vi "enqueue.vi"(6 "priority (f)":bool, 8 "error in (no error)":errorcluster, 9 "data":variant, 10 "cmd":T1, 11 "ComicVine_manager in":refnum<class "ComicVine_manager.lvclass">) -> (0 "error out":errorcluster, 3 "ComicVine_manager out":refnum<class "ComicVine_manager.lvclass">)   [LabVIEW 2024, in "ComicVine_manager.lvclass"]
uses:
  ComicVine_manager.lvclass
  ComicVine_manager.lvclass/ComicVine_manager.ctl
  states--enum.ctl
  queue.message--cluster.ctl
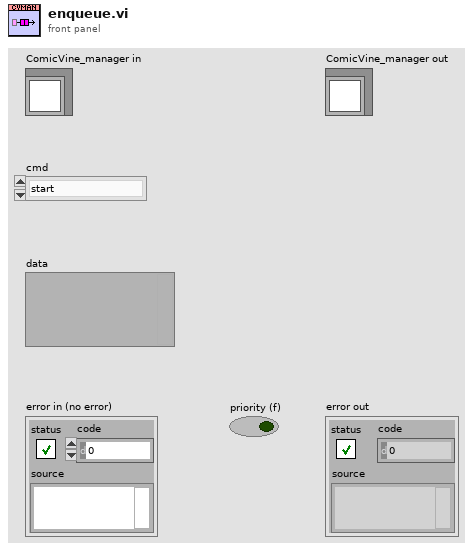
[diagram p1: front panel]
types:
  T1 = typedef "ComicVine_manager.lvclass/states--enum.ctl" = enum16{"start", "running", "shutdown"}
  T2 = typedef "ComicVine_manager.lvclass/queue.message--cluster.ctl" = cluster{"cmd":T1, "data":variant}
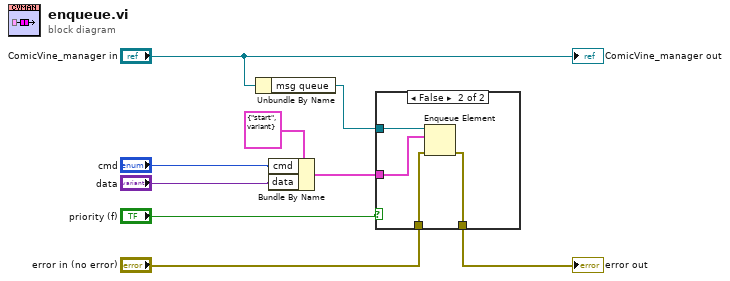
[diagram p0: block diagram]
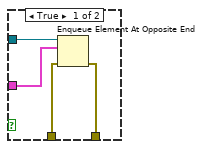
[diagram p2: hidden frame]
diagram:
  n1 = Unbundle By Name("ComicVine_manager in") -> ("msg queue"=w9:refnum<queue>)
  n2 = Bundle By Name(cluster=T2 {"cmd"=enum."start", "data"=variant} ("message"), "cmd"="cmd", "data"="data") -> (w8:T2)
  n3 = case shown="False" "priority (f)" {
    tunnel: w9 -> [w13 w17]
    tunnel: "error in (no error)" -> [w12 w16]
    tunnel: [w11 w15] -> w5
    tunnel: w8 -> [w10 w14]
    frame True {
      n4 = Enqueue Element At Opposite End(queue=w13, element=w10, error in (no error)=w12) -> (error out=w11:errorcluster)  [unwired: 1 in, 2 out]
    }
    frame False {
      n5 = Enqueue Element(queue=w17, element=w14, error in (no error)=w16) -> (error out=w15:errorcluster)  [unwired: 1 in, 2 out]
    }
  }
  "error out" <- w5
  "ComicVine_manager out" <- "ComicVine_manager in"
